vi "About Dialog.vi"(9 "E-mail:":string="smaslan@cmil.cz", 10 "Maintainer:":string="Stanislav Maslan", 11 "Title":string="TWM - Traceable PQ Wattmeter") -> ()   [LabVIEW 2013]
doc: "Shows application about dialog."
uses:
  varilib/varilib.lvlib
panel:
  out "copyright":string="author"
  in  "OK":bool
  out "address":string="Created in scope of the EMPIR project TracePQM.\nDistributed under the MIT license.\n\nAuthors:\n Stanislav Maslan, smaslan@cmi.cz\n Andrei Pokatilov, andrei.pokatilov@metrosert.ee\n \n For authors of the low level instrument drivers see\n readmes in the sourecode."
  out "www:":string="http://www.tracepqm.cmi.cz\nhttps://github.com/smaslan/TWM"
  out "Version:":string
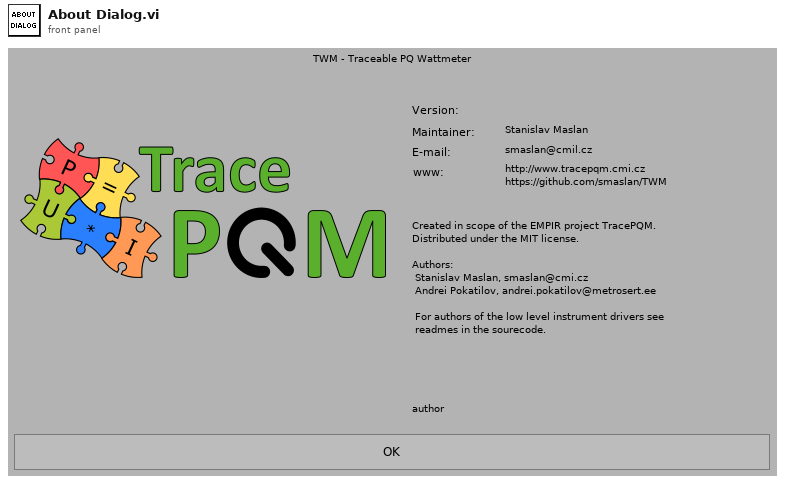
[diagram p1: front panel]
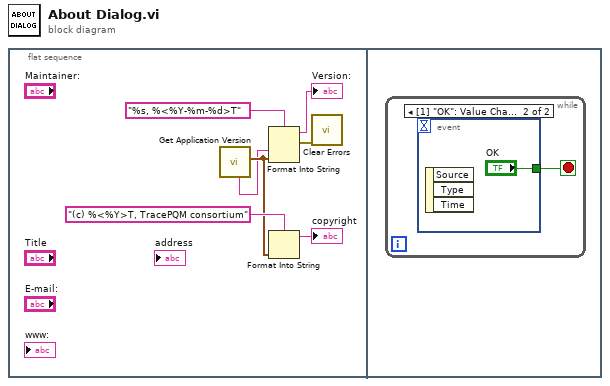
[diagram p0: block diagram]
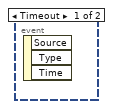
[diagram p2: hidden frame]
diagram:
  n1 = flat-sequence {
    frame #0 {
      n2 = call "Get Application Version.vi"() -> ("last mod"=w2:timestamp, "app. version number"=w1:string)  [unwired: 8 in, 2 out]
      n3 = Format Into String(format string="%s, %<%Y-%m-%d>T" ("time format string (%c)"), w1, w2) -> (resulting string=→"Version:":string, error out=w6:errorcluster)  [unwired: 2 in]
      n4 = Format Into String(format string="(c) %<%Y>T, TracePQM consortium", w2) -> (resulting string=→"copyright":string)  [unwired: 2 in, 1 out]
      n5 = call <vilib>:"Clear Errors.vi"("error in (no error)"=w6) -> ()  [unwired: 6 in, 1 out]
    }
    frame #1 {
      n6 = while {
        stop <- w8 stop-if-true
        n7 = event shown="[1] \"OK\": Value Change;  Panel Close" {
          selector: _ -> [_ _]
          dyn-events: _ -> [_ _]
          timeout: _ -> [_ _]
          tunnel: [_ "OK"] -> w8
          event Timeout {
            n8 = event-data() -> ()  [unwired: 1 in, 3 out]
          }
          event "OK": Value Change; Panel Close {
            n9 = event-data() -> ()  [unwired: 1 in, 3 out]
          }
        }
      }
    }
  }
